vi "saveData.vi"(8 "filename":string="1762scanWithPumping.txt", 10 "dataDirectory":string="c:\\data\\1762 Scans\\") -> (0 "binned path":path=path "c:/data/1762 Scans/2016-08-24-scans/2016-08-24_15-56-18_1762scanWithPumping.txt", 2 "Path":path=path "c:/data/1762 Scans/2016-08-24_15-56-18_1762scanWithPumping.txt")   [LabVIEW 2012]
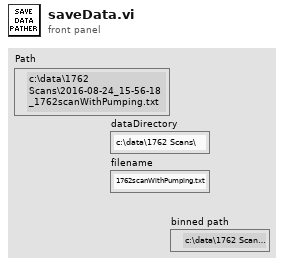
[diagram p1: front panel]
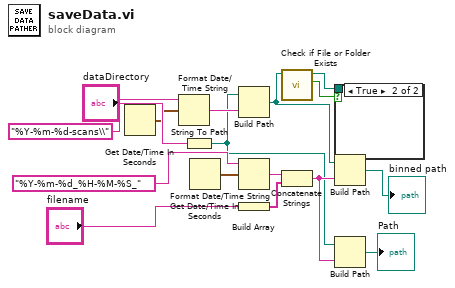
[diagram p0: block diagram]
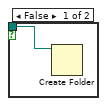
[diagram p2: hidden frame]
diagram:
  n1 = Get Date/Time In Seconds() -> (seconds since 1Jan1904=w9:timestamp)
  n2 = Format Date/Time String(time format string (%c)="%Y-%m-%d-scans\\", seconds (now)=w9) -> (date/time string=w7:string)  [unwired: 1 in]
  n3 = String To Path(string="dataDirectory") -> (path=w4:path)
  n4 = Get Date/Time In Seconds() -> (seconds since 1Jan1904=w12:timestamp)
  n5 = Build Path(base path=w4, name or relative path=w7) -> (appended path=w2:path)
  n6 = Format Date/Time String(time format string (%c)="%Y-%m-%d_%H-%M-%S_", seconds (now)=w12) -> (date/time string=w14:string)  [unwired: 1 in]
  n7 = Build Array("filename") -> (w16:string[])
  n8 = call <vilib>:"Check if File or Folder Exists.vi"("path"=w2) -> ("file or folder exists?"=w3:bool, "dup path"=w1:path)  [unwired: 8 in, 1 out]
  n9 = Concatenate Strings(w14, w16) -> (w6:string)
  n10 = case shown="True" w3 {
    tunnel: w1 -> [w17 _]
    frame False {
      n11 = Create Folder(path (use dialog)=w17) -> ()  [unwired: 2 in, 3 out]
    }
    frame True {
    }
  }
  n12 = Build Path(base path=w2, name or relative path=w6) -> (appended path=→"binned path":path)
  n13 = Build Path(base path=w4, name or relative path=w6) -> (appended path=→"Path":path)
